vi "CleanUp.vi"(0 "reference in":refnum<class "ClassReader.lvclass">, 5 "error in (no error)":errorcluster) -> (14 "reference out":refnum<class "ClassReader.lvclass">, 19 "error out":errorcluster)   [LabVIEW 2020, in "ClassReader.lvclass"]
uses:
  ClassReader.lvclass
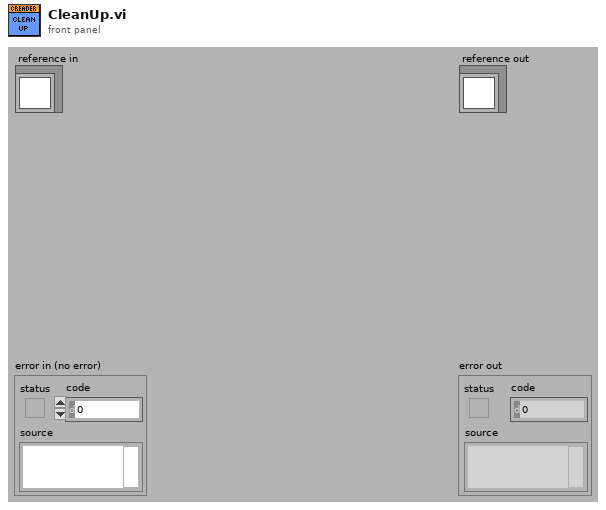
[diagram p1: front panel]
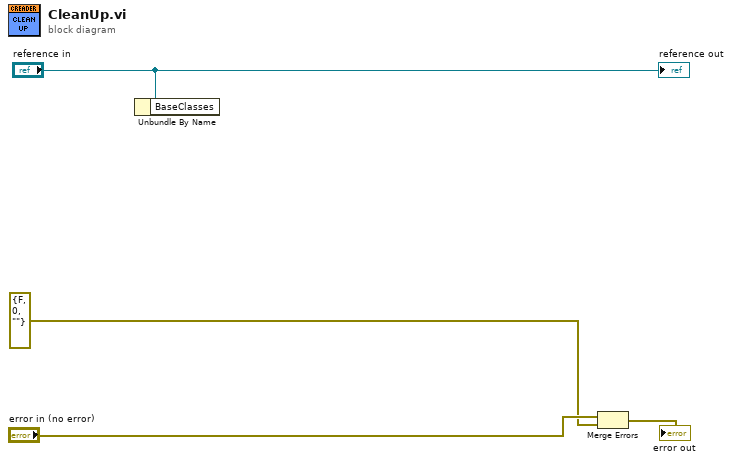
[diagram p0: block diagram]
diagram:
  n1 = Unbundle By Name("reference in") -> ()  [unwired: 1 out]
  n2 = Merge Errors("error in (no error)", errorcluster {"status"=FALSE, "code"=0, "source"=""} ("error in (no error)")) -> (→"error out":errorcluster)
  "reference out" <- "reference in"
